vi "dfd_Super Narrowband Filter Design Masking Filter Create Params.vi"(8 "fstop":dbl, 9 "fpass":dbl, 10 "shaping M":i32) -> (0 "masking original fstop":dbl, 1 "masking original fpass":dbl, 2 "masking N":i32)   [LabVIEW 2017, in "NI_DigFilter_Process.lvlib"]
doc: "Creates the parameters for designing the masking filter."
uses:
  <vilib>/addons/Digital Filter Design/NI_DigFilter_Process.lvlib
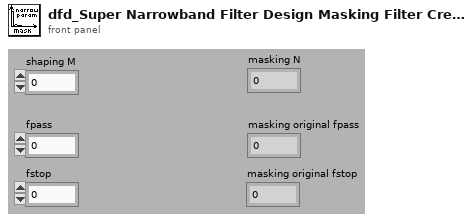
[diagram p1: front panel]
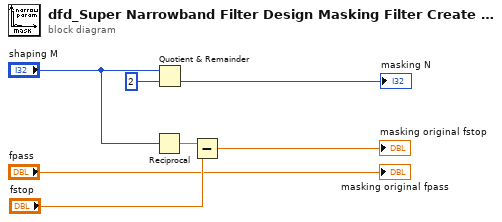
[diagram p0: block diagram]
diagram:
  n1 = Reciprocal(x="shaping M") -> (1/x=w2:dbl)
  n2 = Quotient & Remainder(x="shaping M", y=2) -> (floor(x/y)=→"masking N":i32)  [unwired: 1 out]
  n3 = Subtract(x=w2, y="fstop") -> (x-y=→"masking original fstop":dbl)
  "masking original fpass" <- "fpass"
